vi "GenericJoystickCoerce.vi"(3 "Enable Coercion":bool, 4 "Coerce Limit":dbl=1.0, 5 "Un-Coerced Joystick":dbl) -> (1 "Coerced Joystick":dbl)   [LabVIEW 2020]
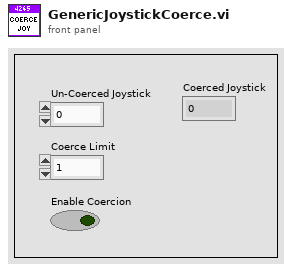
[diagram p1: front panel]
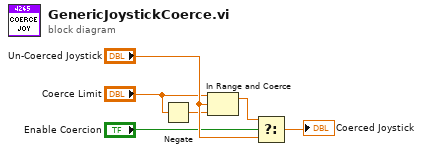
[diagram p0: block diagram]
diagram:
  n1 = Negate(x="Coerce Limit") -> (-x=w3:dbl)
  n2 = In Range and Coerce(upper limit="Coerce Limit", x="Un-Coerced Joystick", lower limit=w3) -> (coerced(x)=w1:dbl)  [unwired: 1 out]
  n3 = Select(t=w1, s="Enable Coercion", f="Un-Coerced Joystick") -> (s? t:f=→"Coerced Joystick":dbl)
